vi "时间格式.vi"() -> (3 "时间格式":T1)   [LabVIEW 2017]
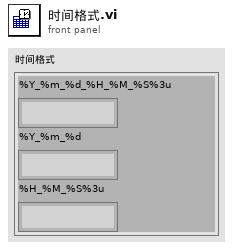
[diagram p1: front panel]
types:
  T1 = cluster{"%Y_%m_%d_%H_%M_%S%3u":string, "%Y_%m_%d":string, "%H_%M_%S%3u":string}
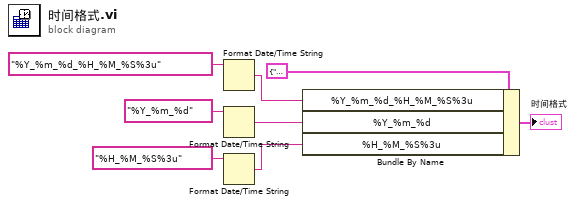
[diagram p0: block diagram]
diagram:
  n1 = Format Date/Time String(time format string (%c)="%Y_%m_%d_%H_%M_%S%3u" ("时间格式字符串(%c)")) -> (date/time string=w5:string)  [unwired: 2 in]
  n2 = Format Date/Time String(time format string (%c)="%Y_%m_%d" ("时间格式字符串(%c)")) -> (date/time string=w6:string)  [unwired: 2 in]
  n3 = Format Date/Time String(time format string (%c)="%H_%M_%S%3u" ("时间格式字符串(%c)")) -> (date/time string=w7:string)  [unwired: 2 in]
  n4 = Bundle By Name(cluster=T1 {"%Y_%m_%d_%H_%M_%S%3u"="", "%Y_%m_%d"="", "%H_%M_%S%3u"=""}, "%Y_%m_%d_%H_%M_%S%3u"=w5, "%Y_%m_%d"=w6, "%H_%M_%S%3u"=w7) -> (→"时间格式":T1)
